vi "Generate file name.vi"(6 "want seconds? (F)":bool, 8 "error in (no error)":errorcluster, 10 "File prefix":string, 11 "Folder Path in":path) -> (0 "error out":errorcluster, 1 "Filename":string, 3 "File Path out":path)   [LabVIEW 2018]
doc: "Generates file name in path base on date and time in Folder\nwith additional prefix nad extension"
panel:
  in  "Extension (txt)":string="txt"
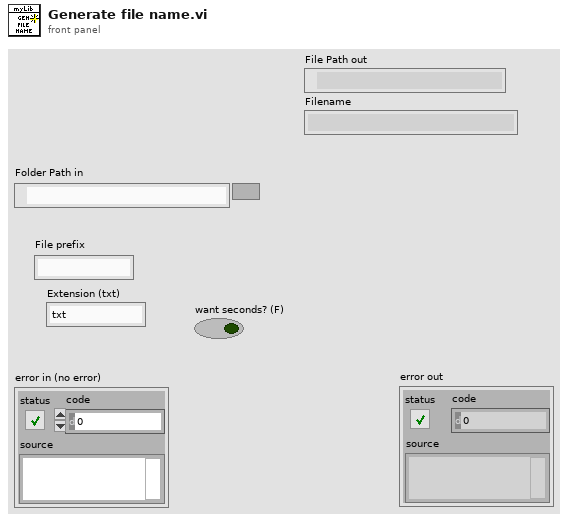
[diagram p1: front panel]
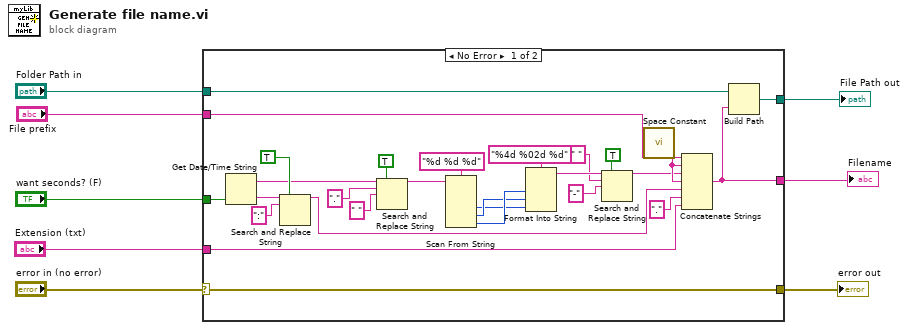
[diagram p0: block diagram]
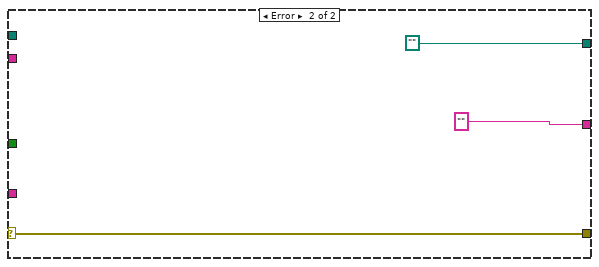
[diagram p2: hidden frame]
diagram:
  n1 = case shown="No Error" "error in (no error)" {
    selector: "error in (no error)" -> [w33 w39]
    tunnel: "want seconds? (F)" -> [w35 _]
    tunnel: [w33 w39] -> w6
    tunnel: "Folder Path in" -> [w32 _]
    tunnel: "File prefix" -> [w31 _]
    tunnel: "Extension (txt)" -> [w28 _]
    tunnel: [w26 path ""] -> w2
    tunnel: [w25 ""] -> w1
    frame No Error {
      n2 = Get Date/Time String(want seconds? (F)=w35) -> (date string=w23:string, time string=w36:string)  [unwired: 2 in]
      n3 = Search and Replace String(replace all?=TRUE ("replace all? (F)"), input string=w36, search string=":") -> (result string=w29:string)  [unwired: 5 in, 3 out]
      n4 = Search and Replace String(replace all?=TRUE ("replace all? (F)"), input string=w23, search string=".", replace string=" " ("replace string (\"\")")) -> (result string=w19:string)  [unwired: 4 in, 3 out]
      n5 = Scan From String(format string="%d %d %d", input string=w19) -> (output 1=w15:i32, output 2=w16:i32, output 3=w17:i32)  [unwired: 5 in, 3 out]
      n6 = Format Into String(format string="%4d %02d %d", w17, w16, w15) -> (resulting string=w13:string)  [unwired: 2 in, 1 out]
      n7 = Search and Replace String(replace all?=TRUE ("replace all? (F)"), input string=w13, search string=" ", replace string="-" ("search string")) -> (result string=w9:string)  [unwired: 4 in, 3 out]
      n8 = call <vilib>:"Space Constant.vi"() -> ("String"=w30:string)
      n9 = Concatenate Strings(w31, w30, w9, w30, w29, "." ("string"), w28) -> (w25:string)
      n10 = Build Path(base path=w32, name or relative path=w25) -> (appended path=w26:path)
    }
    frame Error {
    }
  }
  "error out" <- w6
  "File Path out" <- w2
  "Filename" <- w1
